vi "Safe Mode.vi"(8 "error in (no error)":errorcluster, 11 "Father Of All Detectors in":refnum<class "Father Of All Detectors.lvclass">) -> (0 "error out":errorcluster, 2 "Stop?":bool, 3 "Father Of All Detectors out":refnum<class "Father Of All Detectors.lvclass">)   [LabVIEW 2026, in "TALOS.lvlib" / "Father Of All Detectors.lvlib" / "Father Of All Detectors.lvclass"]
uses:
  Father Of All Detectors.lvclass
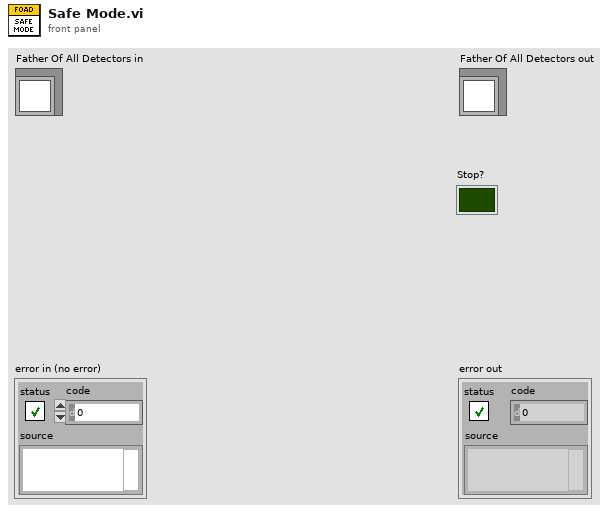
[diagram p1: front panel]
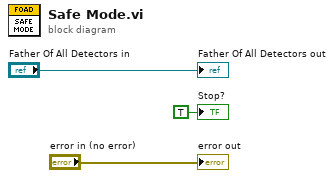
[diagram p0: block diagram]
diagram:
  "error out" <- "error in (no error)"
  "Father Of All Detectors out" <- "Father Of All Detectors in"
  "Stop?" <- TRUE ("Stop?")
